vi "DHE_InterlockMngr.vi"(8 "error in (no error)":errorcluster, 9 "Enum":T2(ring), 10 "command":string) -> (0 "error out":errorcluster, 1 "interlocks":T3(array[cluster]), 2 "response":string, 3 "defined?":bool, 5 "ninter":i32, 7 "states":string[](array[string]))   [LabVIEW 2016]
panel:
  in  "state":T1
  in  "rules":cluster{"command":string, "action":string}
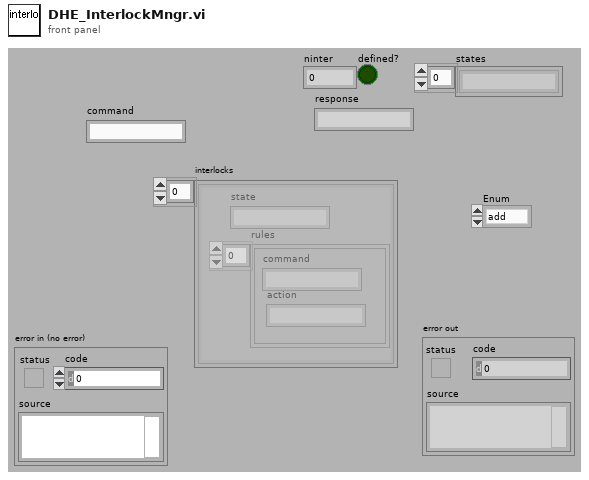
[diagram p1: front panel]
types:
  T1 = cluster{"state":string, "rules":cluster{"command":string, "action":string}[]}
  T2 = enum16{"add", "delete", "find", "clear all", "getall", "all"}
  T3 = cluster{"state":string, "rules":cluster{"command":string, "action":string}[]}[]
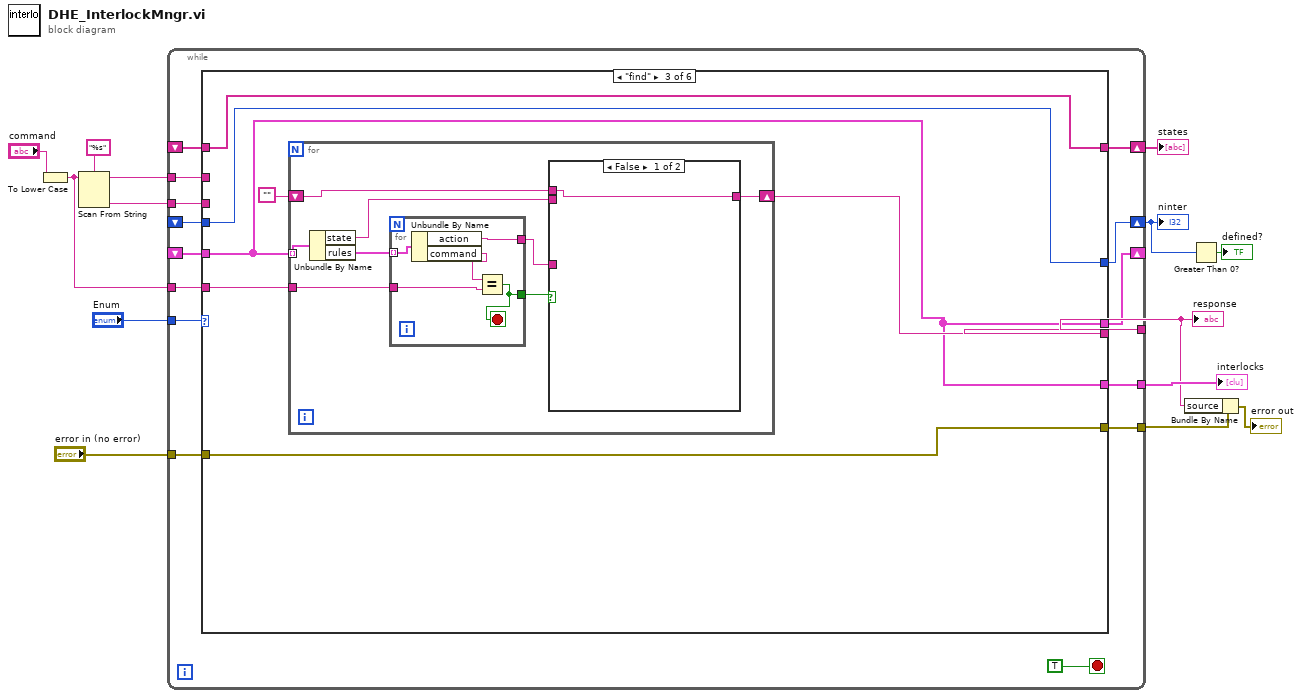
[diagram p0: block diagram]
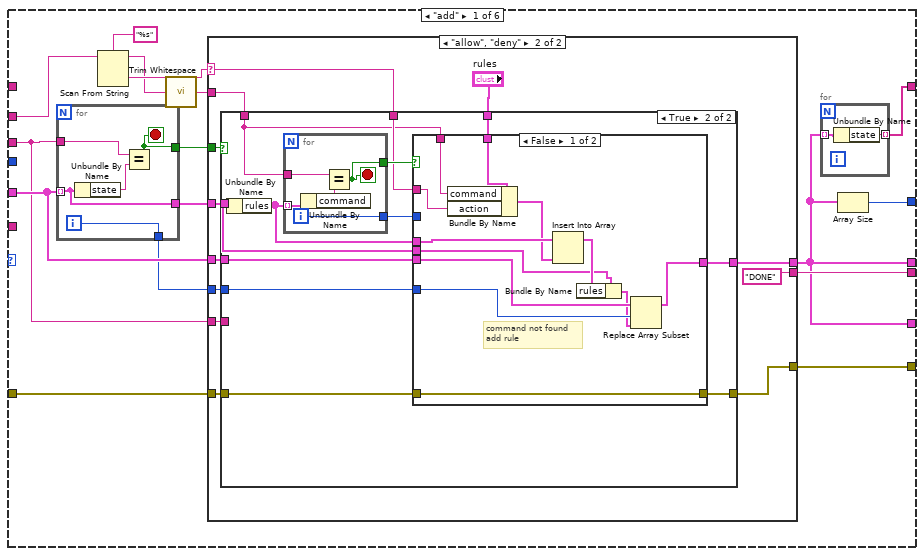
[diagram p2: hidden frame]
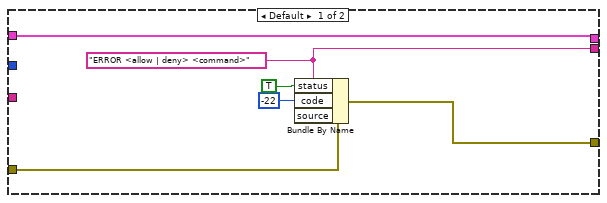
[diagram p3: hidden frame]
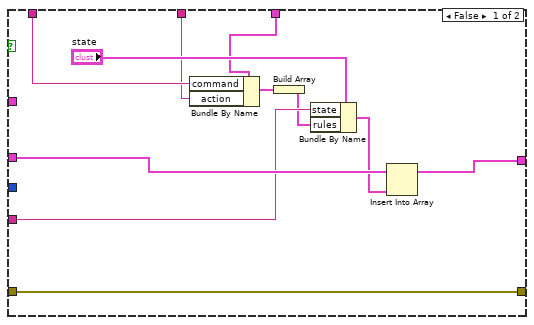
[diagram p4: hidden frame]
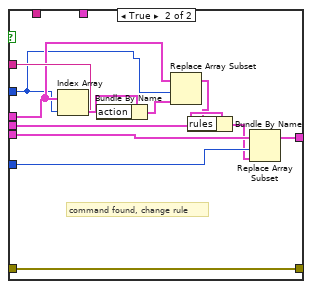
[diagram p5: hidden frame]
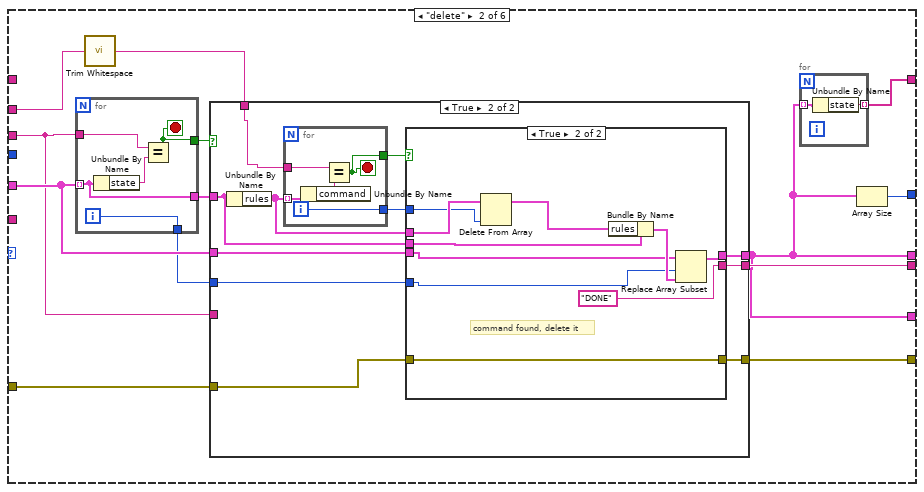
[diagram p6: hidden frame]
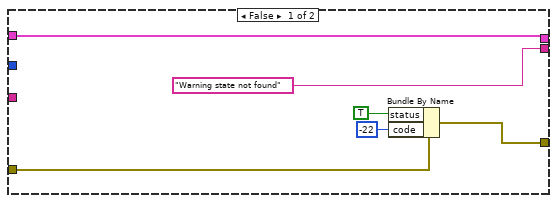
[diagram p7: hidden frame]
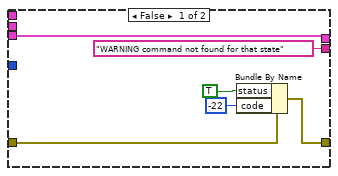
[diagram p8: hidden frame]
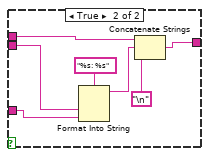
[diagram p9: hidden frame]
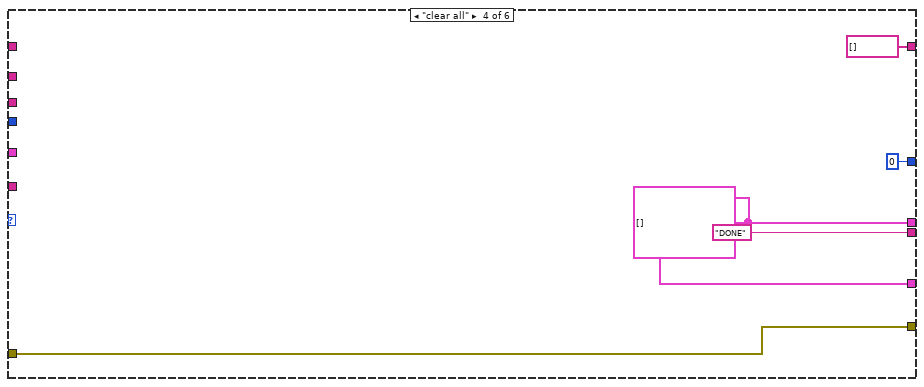
[diagram p10: hidden frame]
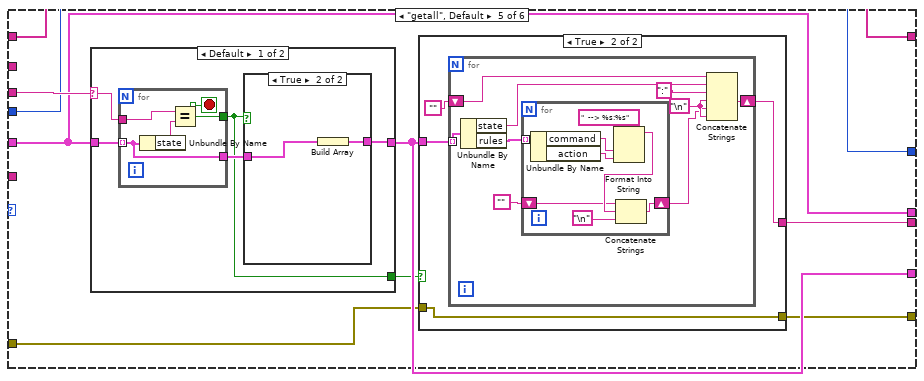
[diagram p11: hidden frame]
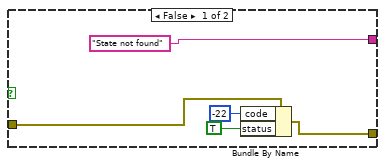
[diagram p12: hidden frame]
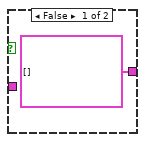
[diagram p13: hidden frame]
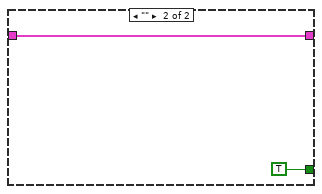
[diagram p14: hidden frame]
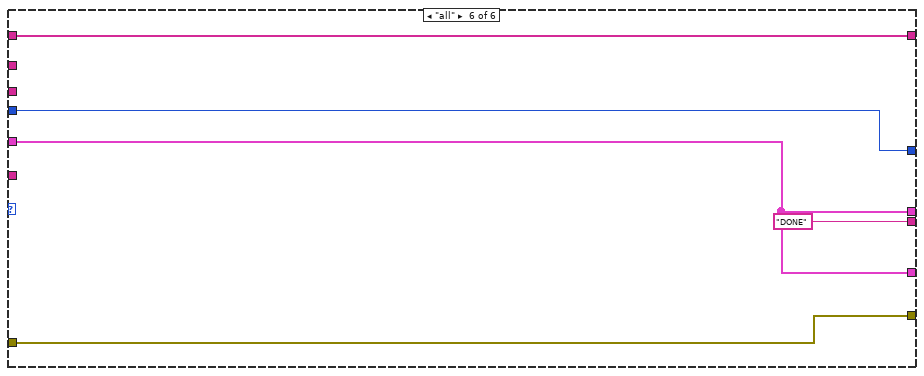
[diagram p15: hidden frame]
diagram:
  n1 = To Lower Case(string="command") -> (all lower case string=w1:string)
  n2 = Scan From String(format string="%s", input string=w1) -> (remaining string=w10:string, output 1=w11:string)  [unwired: 2 in, 3 out]
  n3 = while {
    tunnel: "Enum" -> [w28]
    tunnel: w11 -> [w27]
    tunnel: w10 -> [w26]
    shift-right: [w24] -> _
    shift-left: _ -> [w25]
    tunnel: [w23] -> w7
    tunnel: [w22] -> w9
    tunnel: "error in (no error)" -> [w21]
    tunnel: [w20] -> w6
    shift-right: [w19] -> w4
    shift-left: _ -> [w18]
    shift-right: [w17] -> w3
    shift-left: _ -> [w16]
    tunnel: w1 -> [w15]
    stop <- TRUE stop-if-true
    n4 = case shown="\"find\"" w28 {
      tunnel: w27 -> [w39 w130 _ _ w222 _]
      tunnel: w26 -> [w41 w132 _ _ _ _]
      tunnel: w25 -> [w43 w133 w185 _ w221 w267]
      tunnel: [w33 w125 w185 w212 w221 w267] -> w24
      tunnel: [w38 w129 w186 "DONE" ("response") w218 "DONE" ("response")] -> w23
      tunnel: [w33 w125 w185 w212 w220 w267] -> w22
      tunnel: w21 -> [w37 w128 w184 w211 w217 w266]
      tunnel: [w36 w127 w184 w211 w216 w266] -> w20
      tunnel: [w34 w126 w183 string[] [] w215 w264] -> w19
      tunnel: [w32 w124 w182 0 w214 w263] -> w17
      tunnel: w18 -> [_ _ w183 _ w215 w264]
      tunnel: w16 -> [_ _ w182 _ w214 w263]
      tunnel: w15 -> [_ _ w181 _ _ _]
      frame "add" {
        n5 = for {
          tunnel: w43 -> [w119] mode=indexing
          tunnel: w39 -> [w121]
          tunnel: [w120] -> w45
          tunnel: [w119] -> w44
          tunnel: [w118] -> w40
          i -> [w118]
          stop <- w120 stop-if-true
          n6 = Unbundle By Name(w119) -> ("state"=w122:string)
          n7 = Equal?(x=w121, y=w122) -> (x = y?=w120:bool)
        }
        n8 = Scan From String(format string="%s", input string=w41) -> (remaining string=w31:string, output 1=w35:string)  [unwired: 2 in, 3 out]
        n9 = call <vilib>:"Trim Whitespace.vi"("string"=w31) -> ("trimmed string"=w30:string)  [unwired: 1 in]
        n10 = case shown="\"allow\", \"deny\"" w35 {
          selector: w35 -> [_ w54]
          tunnel: w45 -> [_ w65]
          tunnel: w44 -> [_ w64]
          tunnel: w43 -> [w53 w63]
          tunnel: w30 -> [_ w62]
          tunnel: w40 -> [_ w61]
          tunnel: w39 -> [_ w60]
          tunnel: [w48 "DONE" ("response")] -> w38
          tunnel: [w53 w57] -> w33
          tunnel: w37 -> [w52 w56]
          tunnel: [w51 w55] -> w36
          frame Default {
            w48 = "ERROR <allow | deny> <command>" ("source")
            n11 = Bundle By Name(cluster=w52, "status"=TRUE, "code"=-22, "source"=w48) -> (w51:errorcluster)
          }
          frame "allow", "deny" {
            n12 = case shown="True" w65 {
              tunnel: w64 -> [_ w82]
              tunnel: w63 -> [w76 w87]
              tunnel: w62 -> [w72 w80]
              tunnel: w54 -> [w71 w83]
              tunnel: w61 -> [_ w86]
              tunnel: [w67 w81] -> w57
              tunnel: w60 -> [w74 _]
              tunnel: "rules" -> [w73 w79]
              tunnel: w56 -> [w66 w78]
              tunnel: [w66 w77] -> w55
              frame False {
                n13 = Bundle By Name(cluster=w73, "command"=w72, "action"=w71) -> (w70:cluster{"command":string, "action":string})
                n14 = Build Array(w70) -> (w69:cluster{"command":string, "action":string}[])
                n15 = Bundle By Name(cluster="state", "state"=w74, "rules"=w69) -> (w68:T1)
                n16 = Insert Into Array(array=w76, new element=w68) -> (w67:T3)  [unwired: 1 in]
              }
              frame True {
                n17 = Unbundle By Name(w82) -> ("rules"=w84:cluster{"command":string, "action":string}[])
                n18 = for {
                  tunnel: w84 -> [w117] mode=indexing
                  tunnel: w80 -> [w116]
                  tunnel: [w114] -> w88
                  tunnel: [w113] -> w85
                  i -> [w113]
                  stop <- w114 stop-if-true
                  n19 = Unbundle By Name(w117) -> ("command"=w115:string)
                  n20 = Equal?(x=w116, y=w115) -> (x = y?=w114:bool)
                }
                n21 = case shown="False" w88 {
                  tunnel: w87 -> [w100 w112]
                  tunnel: w86 -> [w96 w111]
                  tunnel: w85 -> [_ w106]
                  tunnel: w84 -> [w95 w107]
                  tunnel: w83 -> [w98 w109]
                  tunnel: w82 -> [w92 w105]
                  tunnel: [w97 w102] -> w81
                  tunnel: w80 -> [w99 _]
                  tunnel: w79 -> [w90 _]
                  tunnel: w78 -> [w89 w101]
                  tunnel: [w89 w101] -> w77
                  frame False {
                    # "command not found\nadd rule"
                    n22 = Bundle By Name(cluster=w90, "command"=w99, "action"=w98) -> (w94:cluster{"command":string, "action":string})
                    n23 = Insert Into Array(array=w95, new element=w94) -> (w93:cluster{"command":string, "action":string}[])  [unwired: 1 in]
                    n24 = Bundle By Name(cluster=w92, "rules"=w93) -> (w91:T1)
                    n25 = Replace Array Subset(array=w100, new element=w91, index=w96) -> (w97:T3)
                  }
                  frame True {
                    # "command found, change rule"
                    n26 = Index Array(array=w107, index=w106) -> (element=w110:cluster{"command":string, "action":string})
                    n27 = Bundle By Name(cluster=w110, "action"=w109) -> (w108:cluster{"command":string, "action":string})
                    n28 = Replace Array Subset(array=w107, new element=w108, index=w106) -> (w104:cluster{"command":string, "action":string}[])
                    n29 = Bundle By Name(cluster=w105, "rules"=w104) -> (w103:T1)
                    n30 = Replace Array Subset(array=w112, new element=w103, index=w111) -> (w102:T3)
                  }
                }
              }
            }
          }
        }
        n31 = for {
          tunnel: w33 -> [w47] mode=indexing
          tunnel: [w46] -> w34 mode=indexing
          n32 = Unbundle By Name(w47) -> ("state"=w46:string)
        }
        n33 = Array Size(array=w33) -> (size(s)=w32:i32)
      }
      frame "delete" {
        n34 = for {
          tunnel: w133 -> [w177] mode=indexing
          tunnel: w130 -> [w179]
          tunnel: [w178] -> w135
          tunnel: [w177] -> w134
          tunnel: [w176] -> w131
          i -> [w176]
          stop <- w178 stop-if-true
          n35 = Unbundle By Name(w177) -> ("state"=w180:string)
          n36 = Equal?(x=w179, y=w180) -> (x = y?=w178:bool)
        }
        n37 = call <vilib>:"Trim Whitespace.vi"("string"=w132) -> ("trimmed string"=w123:string)  [unwired: 1 in]
        n38 = case shown="True" w135 {
          tunnel: w134 -> [_ w147]
          tunnel: w133 -> [w143 w153]
          tunnel: w123 -> [_ w149]
          tunnel: w131 -> [_ w152]
          tunnel: [w143 w150] -> w125
          tunnel: w130 -> [_ _]
          tunnel: ["Warning state not found" ("response") w146] -> w129
          tunnel: w128 -> [w139 w145]
          tunnel: [w138 w144] -> w127
          frame False {
            n39 = Bundle By Name(cluster=w139, "status"=TRUE, "code"=-22) -> (w138:errorcluster)
          }
          frame True {
            n40 = Unbundle By Name(w147) -> ("rules"=w148:cluster{"command":string, "action":string}[])
            n41 = for {
              tunnel: w148 -> [w175] mode=indexing
              tunnel: w149 -> [w174]
              tunnel: [w172] -> w154
              tunnel: [w171] -> w151
              i -> [w171]
              stop <- w172 stop-if-true
              n42 = Unbundle By Name(w175) -> ("command"=w173:string)
              n43 = Equal?(x=w174, y=w173) -> (x = y?=w172:bool)
            }
            n44 = case shown="True" w154 {
              tunnel: w153 -> [w160 w168]
              tunnel: w152 -> [_ w169]
              tunnel: w151 -> [_ w164]
              tunnel: [w160 w167] -> w150
              tunnel: w148 -> [_ w165]
              tunnel: w147 -> [_ w166]
              tunnel: ["WARNING command not found for that state" ("response") "DONE" ("response")] -> w146
              tunnel: w145 -> [w158 w161]
              tunnel: [w157 w161] -> w144
              frame False {
                n45 = Bundle By Name(cluster=w158, "status"=TRUE, "code"=-22) -> (w157:errorcluster)
              }
              frame True {
                # "command found, delete it"
                n46 = Delete From Array(array=w165, index=w164) -> (array with subset deleted=w163:cluster{"command":string, "action":string}[])  [unwired: 1 in, 1 out]
                n47 = Bundle By Name(cluster=w166, "rules"=w163) -> (w170:T1)
                n48 = Replace Array Subset(array=w168, new element=w170, index=w169) -> (w167:T3)
              }
            }
          }
        }
        n49 = for {
          tunnel: w125 -> [w137] mode=indexing
          tunnel: [w136] -> w126 mode=indexing
          n50 = Unbundle By Name(w137) -> ("state"=w136:string)
        }
        n51 = Array Size(array=w125) -> (size(s)=w124:i32)
      }
      frame "find" {
        n52 = for {
          tunnel: w185 -> [w195] mode=indexing
          tunnel: w181 -> [w193]
          shift-right: [w189] -> w186
          shift-left: "" -> [w188]
          n53 = Unbundle By Name(w195) -> ("state"=w190:string, "rules"=w194:cluster{"command":string, "action":string}[])
          n54 = for {
            tunnel: w194 -> [w208] mode=indexing
            tunnel: w193 -> [w206]
            tunnel: [w205] -> w192
            tunnel: [w204] -> w191
            stop <- w205 stop-if-true
            n55 = Unbundle By Name(w208) -> ("action"=w204:string, "command"=w207:string)
            n56 = Equal?(x=w207, y=w206) -> (x = y?=w205:bool)
          }
          n57 = case shown="False" w192 {
            tunnel: w191 -> [_ w201]
            tunnel: w190 -> [_ w202]
            tunnel: [w196 w198] -> w189
            tunnel: w188 -> [w196 w197]
            frame False {
            }
            frame True {
              n58 = Format Into String(format string="%s: %s", w202, w201) -> (resulting string=w200:string)  [unwired: 2 in, 1 out]
              n59 = Concatenate Strings(w197, w200, "\n") -> (w198:string)
            }
          }
        }
      }
      frame "clear all" {
        w212 = T3 []
      }
      frame "getall", Default {
        n60 = case shown="Default" w222 {
          selector: w222 -> [w252 _]
          tunnel: w221 -> [w253 w262]
          tunnel: [w250 w262] -> w220
          tunnel: [w249 TRUE] -> w219
          frame Default {
            n61 = for {
              tunnel: w253 -> [w257] mode=indexing
              tunnel: w252 -> [w259]
              tunnel: [w258] -> w249
              tunnel: [w257] -> w251
              stop <- w258 stop-if-true
              n62 = Unbundle By Name(w257) -> ("state"=w260:string)
              n63 = Equal?(x=w259, y=w260) -> (x = y?=w258:bool)
            }
            n64 = case shown="True" w249 {
              tunnel: w251 -> [_ w256]
              tunnel: [T3 [] w255] -> w250
              frame False {
              }
              frame True {
                n65 = Build Array(w256) -> (w255:T3)
              }
            }
          }
          frame "" {
          }
        }
        n66 = case shown="True" w219 {
          tunnel: w220 -> [_ w231]
          tunnel: ["State not found" ("response") w229] -> w218
          tunnel: w217 -> [w226 w228]
          tunnel: [w224 w228] -> w216
          frame False {
            n67 = Bundle By Name(cluster=w226, "code"=-22, "status"=TRUE) -> (w224:errorcluster)
          }
          frame True {
            n68 = for {
              tunnel: w231 -> [w240] mode=indexing
              shift-right: [w234] -> w229
              shift-left: "" -> [w237]
              w233 = "\n"
              n69 = Unbundle By Name(w240) -> ("state"=w236:string, "rules"=w239:cluster{"command":string, "action":string}[])
              n70 = for {
                tunnel: w239 -> [w248] mode=indexing
                shift-right: [w243] -> w232
                shift-left: "" -> [w242]
                n71 = Unbundle By Name(w248) -> ("command"=w247:string, "action"=w246:string)
                n72 = Format Into String(format string="  --> %s:%s", w247, w246) -> (resulting string=w244:string)  [unwired: 2 in, 1 out]
                n73 = Concatenate Strings(w242, w244, "\n") -> (w243:string)
              }
              n74 = Concatenate Strings(w237, w236, ":" ("string"), w233, w232, w233) -> (w234:string)
            }
          }
        }
      }
      frame "all" {
      }
    }
  }
  "response" <- w7
  "interlocks" <- w9
  "states" <- w4
  "ninter" <- w3
  n75 = Bundle By Name(cluster=w6, "source"=w7) -> (→"error out":errorcluster)
  n76 = Greater Than 0?(x=w3) -> (x > 0?=→"defined?":bool)
